vi "SystemSearchDataName.vi"(11 "element":string) -> (1 "Index":cluster{"Y":i32, "X":i32}, 2 "variant":variant, 3 "DataOut":string)   [LabVIEW 2019]
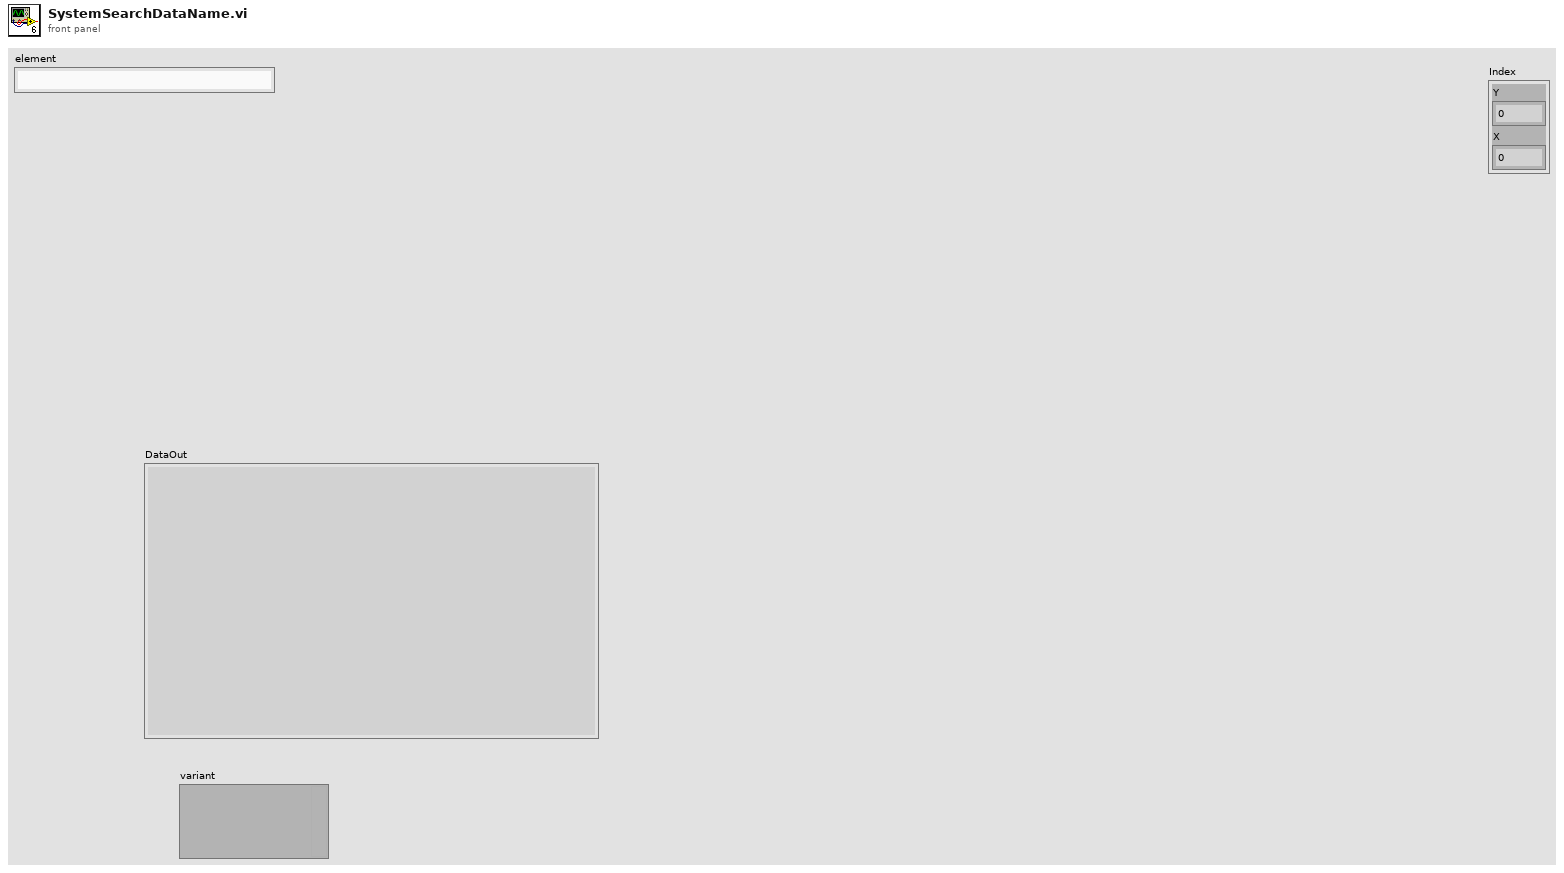
[diagram p1: front panel]
types:
  T1 = cluster{"type string":i16[], "data string":string}
  T2 = enum16{"initial", "save", "load", "write", "read"}
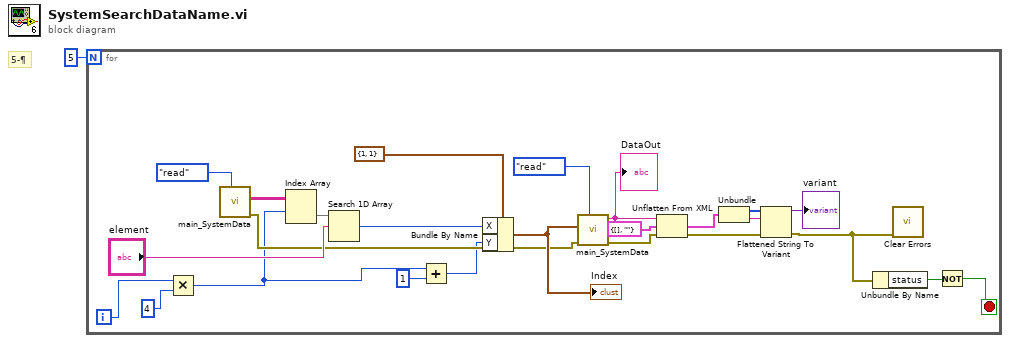
[diagram p0: block diagram]
diagram:
  # "5­¶"
  n1 = for {
    N: 5 -> [_]
    i -> [w8]
    stop <- w6 stop-if-true
    n2 = Multiply(x=w8, y=4) -> (x*y=w4:i32)
    n3 = call "main_SystemData.vi"("Enum"=T2."read") -> ("error out"=w12:errorcluster, "Table Control"=w21:string[][])  [unwired: 8 in, 1 out]
    n4 = Index Array(array=w21, index (row)=w4) -> (element=w22:string[])  [unwired: 1 in]
    n5 = Search 1D Array(1D array=w22, element="element") -> (index of element=w5:i32)  [unwired: 1 in]
    n6 = Add(x=w4, y=1) -> (x+y=w2:i32)
    n7 = Bundle By Name(cluster=cluster{"Y":i32, "X":i32} {"Y"=1, "X"=1} ("Index"), "X"=w5, "Y"=w2) -> (w26:cluster{"Y":i32, "X":i32})
    "Index" <- w26
    n8 = call "main_SystemData.vi"("Enum"=T2."read", "error in"=w12, "Index"=w26) -> ("error out"=w11:errorcluster, "DataOut"=w14:string)  [unwired: 6 in, 1 out]
    "DataOut" <- w14
    n9 = Unflatten From XML(xml string=w14, type=T1 {"type string"=[], "data string"=""} ("cluster"), error in (no error)=w11) -> (value=w18:T1, error out=w15:errorcluster)
    n10 = Unbundle(w18) -> ("type string"=w17:i16[], "data string"=w16:string)
    n11 = Flattened String To Variant(4:w15, 6:w16, 7:w17) -> (0:w10:errorcluster, 3:→"variant":variant)
    n12 = Unbundle By Name(w10) -> ("status"=w9:bool)
    n13 = call <vilib>:"Clear Errors.vi"("error in (no error)"=w10) -> ()  [unwired: 5 in, 2 out]
    n14 = Not(x=w9) -> (.not. x?=w6:bool)
  }
